vi "S2DS_Add single WC.vi"(4 "WC Present value":dbl, 6 "WC Factor":dbl, 7 "WC instrument menu":string, 10 "WC name in":string, 11 "prefix":string) -> (0 "Write channel info":T1, 1 "WC name out":string, 2 "Prefix":string, 5 "Base unit":string)   [LabVIEW 2025]
uses:
  TYPE DEFS/S2DS_Single WC info.ctl
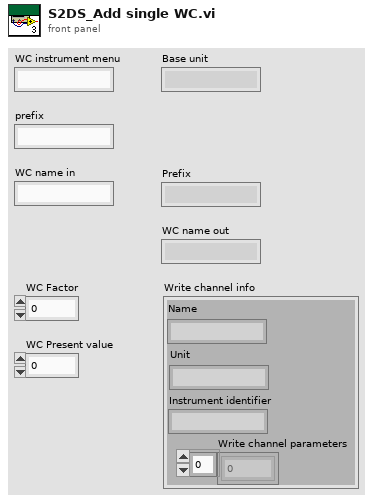
[diagram p1: front panel]
types:
  T1 = typedef "S2DS_Single WC info.ctl" = cluster{"Instrument identifier":string, "Write channel parameters":dbl[], "Name":string, "Unit":string}
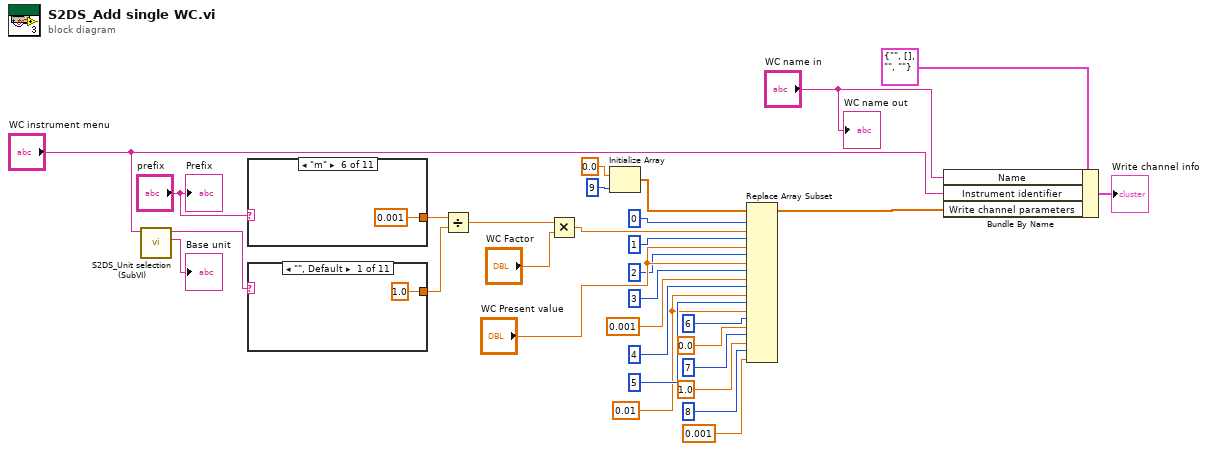
[diagram p0: block diagram]
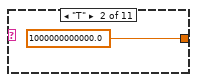
[diagram p2: hidden frame]
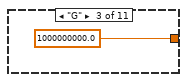
[diagram p3: hidden frame]
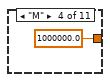
[diagram p4: hidden frame]
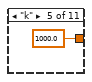
[diagram p5: hidden frame]
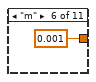
[diagram p6: hidden frame]
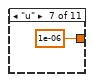
[diagram p7: hidden frame]
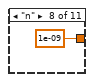
[diagram p8: hidden frame]
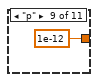
[diagram p9: hidden frame]
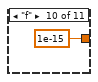
[diagram p10: hidden frame]
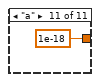
[diagram p11: hidden frame]
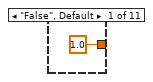
[diagram p12: hidden frame]
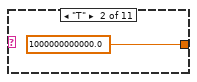
[diagram p13: hidden frame]
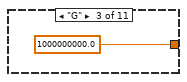
[diagram p14: hidden frame]
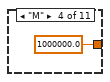
[diagram p15: hidden frame]
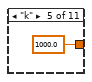
[diagram p16: hidden frame]
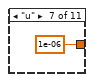
[diagram p17: hidden frame]
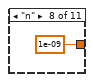
[diagram p18: hidden frame]
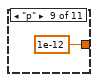
[diagram p19: hidden frame]
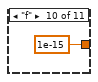
[diagram p20: hidden frame]
diagram:
  w17 = 0.01
  n1 = call "S2DS_Unit selection (SubVI).vi"("RC instrument name"="WC instrument menu") -> ("Base unit"=→"Base unit":string, "Instrument default prefix"=w9:string)  [unwired: 9 in]
  n2 = case shown="\"m\"" "prefix" {
    tunnel: [1.0 1000000000000.0 1000000000.0 1000000.0 1000.0 0.001 1e-06 1e-09 1e-12 1e-15 1e-18] -> w14
    frame "False", Default {
    }
    frame "T" {
    }
    frame "G" {
    }
    frame "M" {
    }
    frame "k" {
    }
    frame "m" {
    }
    frame "u" {
    }
    frame "n" {
    }
    frame "p" {
    }
    frame "f" {
    }
    frame "a" {
    }
  }
  n3 = case shown="\"\", Default" w9 {
    tunnel: [1.0 1000000000000.0 1000000000.0 1000000.0 1000.0 0.001 1e-06 1e-09 1e-12 1e-15 1e-18] -> w13
    frame "", Default {
    }
    frame "T" {
    }
    frame "G" {
    }
    frame "M" {
    }
    frame "k" {
    }
    frame "m" {
    }
    frame "u" {
    }
    frame "n" {
    }
    frame "p" {
    }
    frame "f" {
    }
    frame "a" {
    }
  }
  n4 = Divide(x=w14, y=w13) -> (x/y=w16:dbl)
  n5 = Multiply(x=w16, y="WC Factor") -> (x*y=w15:dbl)
  n6 = Initialize Array(0.0 ("element"), 9 ("dimension size")) -> (w22:dbl[])
  n7 = Replace Array Subset(array=w22, new element #1=w15, index #1=0 ("index"), new element #2="WC Present value", index #2=1 ("index"), new element #3="WC Present value", index #3=2 ("index"), new element #4=0.001, index #4=3 ("index"), new element #5=w17, index #5=4 ("index"), new element #6=w17, index #6=5 ("index"), new element #7=0.0 ("new element/subarray"), index #7=6 ("index"), new element #8=1.0 ("new element/subarray"), index #8=7 ("index"), new element #9=0.001 ("new element/subarray"), index #9=8 ("index")) -> (w28:dbl[])
  n8 = Bundle By Name(cluster=T1 {"Instrument identifier"="", "Write channel parameters"=[], "Name"="", "Unit"=""} ("Write channel info 2"), "Name"="WC name in", "Instrument identifier"="WC instrument menu", "Write channel parameters"=w28) -> (→"Write channel info":T1)
  "WC name out" <- "WC name in"
  "Prefix" <- "prefix"
